vi "Set Maximum Data Duration.vi"(9 "maximum data duration":dbl=-1.0, 11 "variant in":variant) -> (3 "variant out":variant)   [LabVIEW 2017]
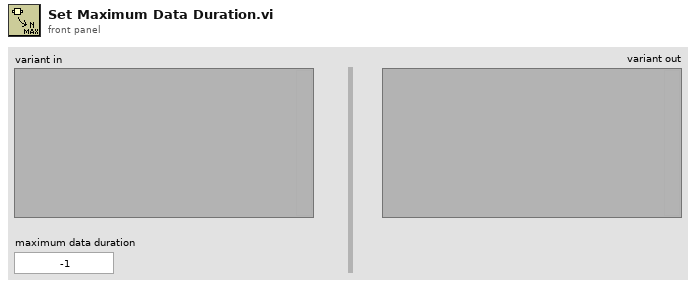
[diagram p1: front panel]
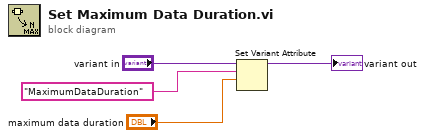
[diagram p0: block diagram]
diagram:
  n1 = Set Variant Attribute(Variant="variant in", name="MaximumDataDuration", value="maximum data duration") -> (Variant out=→"variant out":variant)  [unwired: 1 in, 2 out]
